vi "Read xCorrection_arcsec.vi"(8 "error in (no error)":errorcluster, 11 "AOSPointingOffset in":refnum<class "AOSPointingOffset.lvclass">) -> (0 "error out":errorcluster, 2 "xCorrection_arcsec":dbl[unit] min=-0.001454441043328608 max=0.001454441043328608, 3 "AOSPointingOffset out":refnum<class "AOSPointingOffset.lvclass">)   [LabVIEW 2014, in "TCSDataDefinitions.lvlib" / "TCSActiveOpticsCommand.lvlib" / "AOSPointingOffset.lvclass"]
uses:
  AOSPointingOffset.lvclass
  AOSPointingOffset.lvclass/AOSPointingOffset.ctl
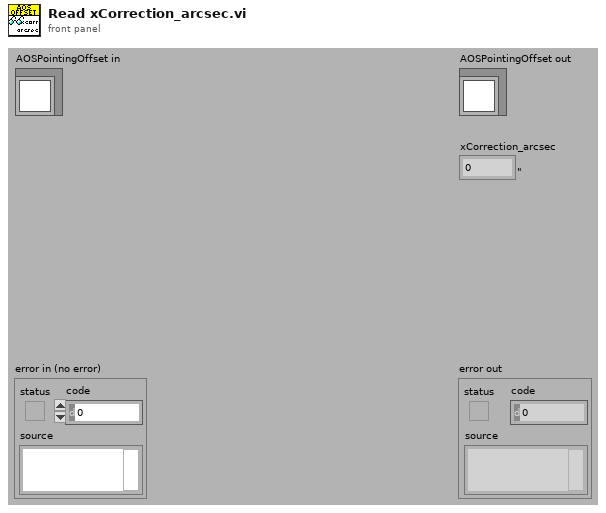
[diagram p1: front panel]
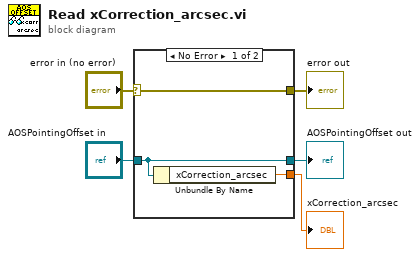
[diagram p0: block diagram]
diagram:
  n1 = case shown="No Error" "error in (no error)" {
    selector: "error in (no error)" -> [w8 w9]
    tunnel: [w8 w9] -> w4
    tunnel: [w7 w10] -> w2
    tunnel: "AOSPointingOffset in" -> [w7 w10]
    tunnel: [w6 _] -> w1
    frame No Error {
      n2 = Unbundle By Name(w7) -> ("xCorrection_arcsec"=w6:dbl[unit])
    }
    frame Error {
    }
  }
  "error out" <- w4
  "AOSPointingOffset out" <- w2
  "xCorrection_arcsec" <- w1
